vi "Write Setpoint.vi"(8 "error in":errorcluster, 10 "Setpoint":sgl, 11 "Alicat Device in":refnum<class "Alicat Device.lvclass">) -> (0 "error out":errorcluster, 2 "DataOut":string, 3 "Alicat Device out":refnum<class "Alicat Device.lvclass">)   [LabVIEW 2019, in "Alicat Device.lvclass"]
doc: "Send a command to the controller for the setpoint. The command will be in the format <b>Xnnnnn</b> where <b>X</b> is the address and <b>nnnnn</b> is a setpoint value that ranges from 0 to 64000. The setpoint is based on the <b>Fullscale</b> value and can be calculated as\n\nnnnnn = SP*64000/FS\n\nWhen the command for a new setpoint is sent, the controller will respond with the current data values. The input <b>Setpoint</b> will be coerced in the range 0 to Full Scale."
uses:
  Alicat Device.lvclass
  Alicat Device.lvclass/Alicat Device.ctl
  Reusable/Session APIs/Serial/Public/Get Data/Get String.vi
  Reusable/Session APIs/Text Communication/Text Device Session.lvclass
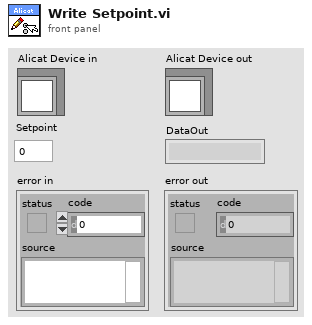
[diagram p1: front panel]
types:
  T1 = typedef "Session - Root.lvclass/Session Handle.ctl" = refnum<data-value>
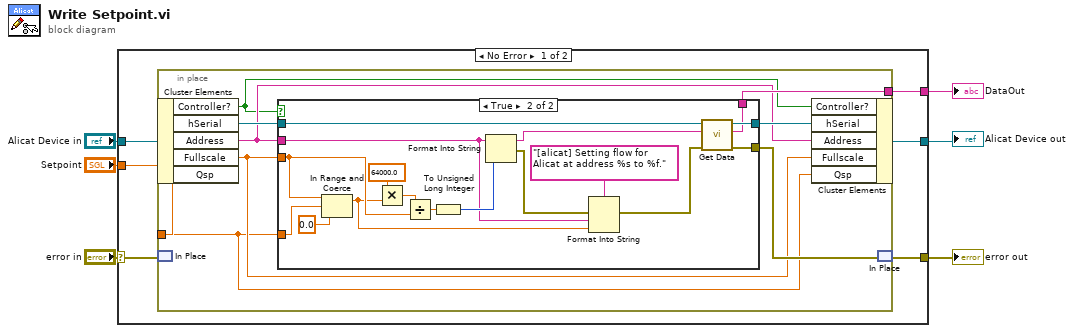
[diagram p0: block diagram]
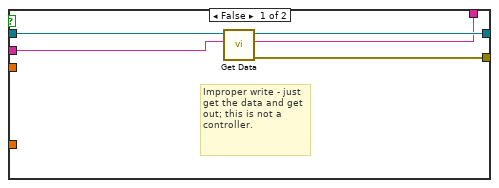
[diagram p2: hidden frame]
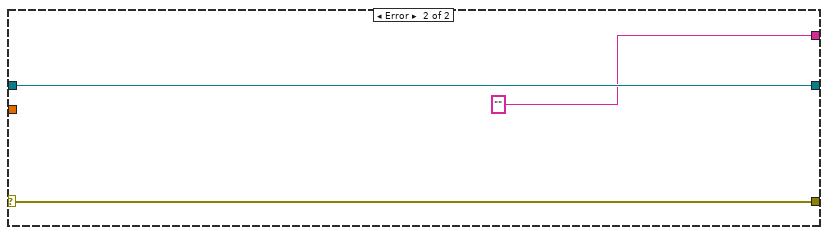
[diagram p3: hidden frame]
diagram:
  n1 = case shown="No Error" "error in" {
    selector: "error in" -> [w11 w45]
    tunnel: "Alicat Device in" -> [w12 w44]
    tunnel: [w9 w45] -> w2
    tunnel: [w10 w44] -> w3
    tunnel: [w8 "" ("DataOut")] -> w4
    tunnel: "Setpoint" -> [w7 _]
    frame No Error {
      n2 = in-place {
        in-place-border: [w17] -> w8
        in-place-border: w7 -> [w13]
        n3 = in-place-cluster #1(w12) -> ("Controller?"=w14:bool, "hSerial"=w20:T1, "Address"=w16:string, "Fullscale"=w15:sgl)  [unwired: 1 out]
        n4 = in-place-match #2(w11) -> ()  [unwired: 1 out]
        n5 = case shown="True" w14 {
          tunnel: w20 -> [w24 w42]
          tunnel: [w23 w41] -> w19
          tunnel: [w21 w28] -> w18
          tunnel: [w22 w40] -> w17
          tunnel: w16 -> [w25 w31]
          tunnel: w15 -> [_ w34]
          tunnel: w13 -> [_ w32]
          frame False {
            # "Improper write - just get the data and get out; this is not a controller."
            n6 = call-poly "Get Data.vi"("CMD"=w25, "handle in"=w24) -> ("error out"=w21:errorcluster, "DataOut"=w22:string, "handle out"=w23:T1)  [unwired: 7 in]
          }
          frame True {
            n7 = In Range and Coerce(upper limit=w34, x=w32, lower limit=sgl 0.0) -> (coerced(x)=w29:sgl)  [unwired: 1 out]
            n8 = Multiply(x=sgl 64000.0, y=w29) -> (x*y=w38:sgl)
            n9 = Divide(x=w38, y=w34) -> (x/y=w37:sgl)
            n10 = To Unsigned Long Integer(number=w37) -> (unsigned 32bit integer=w35:u32)
            n11 = Format Into String(initial string=w31, w35) -> (resulting string=w39:string, error out=w26:errorcluster)  [unwired: 2 in]
            n12 = Format Into String(format string="[alicat] Setting flow for Alicat at address %s to %f.", error in=w26, w31, w29) -> (error out=w27:errorcluster)  [unwired: 1 in, 1 out]
            n13 = call-poly "Get Data.vi"("error in"=w27, "CMD"=w39, "handle in"=w42) -> ("error out"=w28:errorcluster, "DataOut"=w40:string, "handle out"=w41:T1)  [unwired: 6 in]
          }
        }
        n14 = in-place-cluster #1("Controller?"=w14, "hSerial"=w19, "Address"=w16, "Fullscale"=w15, "Qsp"=w13) -> (w10:refnum<class "Alicat Device.lvclass">)
        n15 = in-place-match #2(w18) -> (w9:errorcluster)
      }
    }
    frame Error {
    }
  }
  "error out" <- w2
  "Alicat Device out" <- w3
  "DataOut" <- w4
